vi "CMD_COMPOSE.vi"(6 "Gantry in":refnum<class "Gantry.lvclass">, 8 "error in (no error)":errorcluster, 10 "Arguments":string[](array[string]), 11 "gScript Interpreter in":refnum<class "gScript Interpreter.lvclass">) -> (0 "error out":errorcluster, 3 "gScript Interpreter out":refnum<class "gScript Interpreter.lvclass">, 4 "Gantry out":refnum<class "Gantry.lvclass">)   [LabVIEW 2023, in "gScript Interpreter.lvclass"]
uses:
  gScript Interpreter.lvclass
  Shared Components/Gantry Class/Gantry.lvclass
  Type Definitions/Memory Cell Type Enum.ctl
  Shared Components/Orient3d Class/Orient3d.lvclass
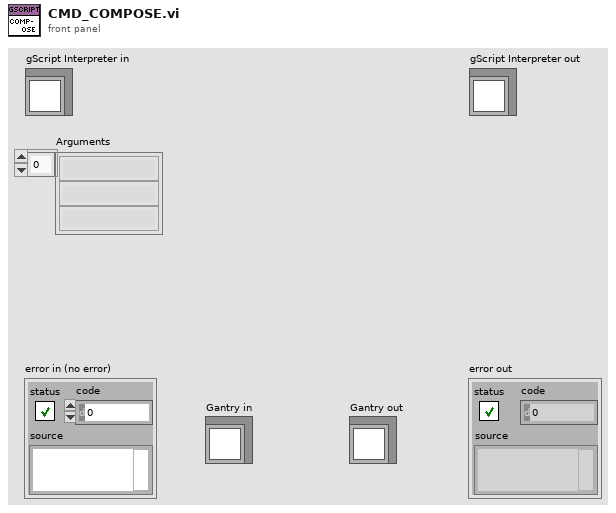
[diagram p1: front panel]
types:
  T1 = typedef "Memory Cell Type Enum.ctl" = enum16{"integer", "float", "vector", "rotation"}
  T2 = typedef "Memory Cell.ctl" = cluster{"type":T1, "x":dbl, "y":dbl, "z":dbl, "w":dbl}
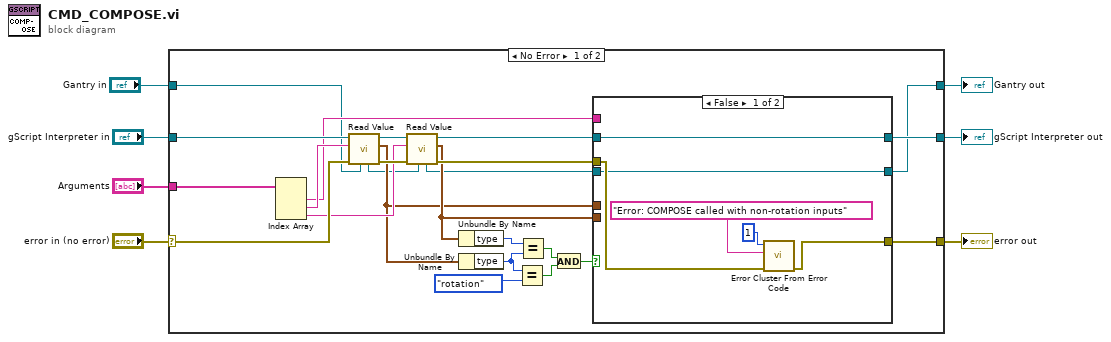
[diagram p0: block diagram]
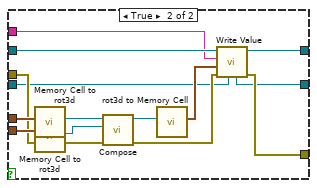
[diagram p2: hidden frame]
diagram:
  n1 = case shown="No Error" "error in (no error)" {
    selector: "error in (no error)" -> [w29 w54]
    tunnel: [w20 w54] -> w6
    tunnel: [w21 w53] -> w4
    tunnel: "gScript Interpreter in" -> [w30 w53]
    tunnel: "Arguments" -> [w31 _]
    tunnel: "Gantry in" -> [w11 w52]
    tunnel: [w8 w52] -> w1
    frame No Error {
      n2 = Index Array(array=w31) -> (element #1=w23:string, element #2=w28:string, element #3=w25:string)  [unwired: 3 in]
      n3 = call-dynamic "Read Value.vi"("Gantry in"=w11, "error in (no error)"=w29, "String in"=w28, "gScript Interpreter in"=w30) -> ("error out"=w27:errorcluster, "Memory Cell"=w12:T2, "gScript Interpreter out"=w26:refnum<class "gScript Interpreter.lvclass">, "Gantry out"=w10:refnum<class "Gantry.lvclass">)  [unwired: 4 in]
      n4 = call-dynamic "Read Value.vi"("Gantry in"=w10, "error in (no error)"=w27, "String in"=w25, "gScript Interpreter in"=w26) -> ("error out"=w22:errorcluster, "Memory Cell"=w13:T2, "gScript Interpreter out"=w24:refnum<class "gScript Interpreter.lvclass">, "Gantry out"=w9:refnum<class "Gantry.lvclass">)  [unwired: 4 in]
      n5 = Unbundle By Name(w13) -> ("type"=w19:T1)
      n6 = Unbundle By Name(w12) -> ("type"=w18:T1)
      n7 = Equal?(x=w18, y=Memory_Cell_Type_Enum."rotation" ("Memory Cell Type Enum")) -> (x = y?=w15:bool)
      n8 = Equal?(x=w19, y=w18) -> (x = y?=w16:bool)
      n9 = And(x=w16, y=w15) -> (x .and. y?=w14:bool)
      n10 = case shown="False" w14 {
        tunnel: w24 -> [w37 w51]
        tunnel: w23 -> [_ w50]
        tunnel: w22 -> [w34 w43]
        tunnel: [w37 w49] -> w21
        tunnel: [w33 w48] -> w20
        tunnel: w13 -> [_ w46]
        tunnel: w12 -> [_ w47]
        tunnel: w9 -> [w32 w39]
        tunnel: [w32 w38] -> w8
        frame False {
          n11 = call <vilib>:"Error Cluster From Error Code.vi"("error in (no error)"=w34, "error message (\"\")"="Error: COMPOSE called with non-rotation inputs" ("error message (\"\")"), "error code (0)"=1) -> ("error out"=w33:errorcluster)  [unwired: 6 in]
        }
        frame True {
          n12 = call "Memory Cell to rot3d.vi"("Memory Cell"=w47) -> ("Orient3d out"=w45:refnum<class "Orient3d.lvclass">)  [unwired: 10 in]
          n13 = call "Memory Cell to rot3d.vi"("Memory Cell"=w46) -> ("Orient3d out"=w44:refnum<class "Orient3d.lvclass">)  [unwired: 10 in]
          n14 = call "Compose.vi"("error in"=w43, "Orient3d 2"=w44, "Orient3d 1"=w45) -> ("error out"=w42:errorcluster, "Orient3d out"=w41:refnum<class "Orient3d.lvclass">)  [unwired: 7 in]
          n15 = call "rot3d to Memory Cell.vi"("Orient3d in"=w41) -> ("Memory Cell"=w40:T2)  [unwired: 10 in]
          n16 = call-dynamic "Write Value.vi"("Gantry in"=w39, "error in (no error)"=w42, "Value"=w40, "Address"=w50, "gScript Interpreter in"=w51) -> ("error out"=w48:errorcluster, "gScript Interpreter out"=w49:refnum<class "gScript Interpreter.lvclass">, "Gantry out"=w38:refnum<class "Gantry.lvclass">)  [unwired: 4 in]
        }
      }
    }
    frame Error {
    }
  }
  "error out" <- w6
  "gScript Interpreter out" <- w4
  "Gantry out" <- w1
